vi "Distance Conversion.vi"() -> ()   [LabVIEW 2015]
uses:
  Distance Unit.ctl
panel:
  out "Output Distance":dbl
  in  "Output Unit":T1
  in  "Input Unit":T1
  in  "Input Distance":dbl
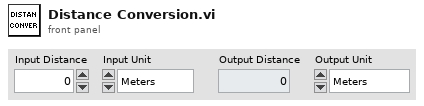
[diagram p1: front panel]
types:
  T1 = typedef "Distance Unit.ctl" = enum16{"Meters", "Miles", "Kilometers", "Yards"}
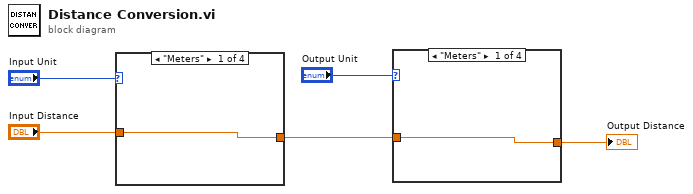
[diagram p0: block diagram]
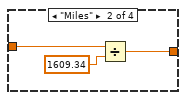
[diagram p2: hidden frame]
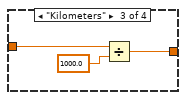
[diagram p3: hidden frame]
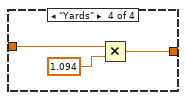
[diagram p4: hidden frame]
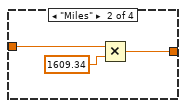
[diagram p5: hidden frame]
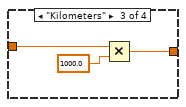
[diagram p6: hidden frame]
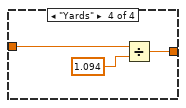
[diagram p7: hidden frame]
diagram:
  n1 = case shown="\"Meters\"" "Input Unit" {
    tunnel: "Input Distance" -> [w6 w9 w12 w15]
    tunnel: [w6 w7 w10 w13] -> w2
    frame "Meters" {
    }
    frame "Miles" {
      n2 = Multiply(x=w9, y=1609.34) -> (x*y=w7:dbl)
    }
    frame "Kilometers" {
      n3 = Multiply(x=w12, y=1000.0) -> (x*y=w10:dbl)
    }
    frame "Yards" {
      n4 = Divide(x=w15, y=1.094) -> (x/y=w13:dbl)
    }
  }
  n5 = case shown="\"Meters\"" "Output Unit" {
    tunnel: w2 -> [w16 w19 w22 w25]
    tunnel: [w16 w17 w20 w23] -> w1
    frame "Meters" {
    }
    frame "Miles" {
      n6 = Divide(x=w19, y=1609.34) -> (x/y=w17:dbl)
    }
    frame "Kilometers" {
      n7 = Divide(x=w22, y=1000.0) -> (x/y=w20:dbl)
    }
    frame "Yards" {
      n8 = Multiply(x=w25, y=1.094) -> (x*y=w23:dbl)
    }
  }
  "Output Distance" <- w1
